vi "multitest.vi"   [LabVIEW 2015, in "SystemLink File Module tests.lvlib"]
uses:
  SystemLink File Module tests.lvlib
  module/configuration/SystemLink File configuration.lvclass
  <vilib>/Skyline/Tag/Wrapper/Wrapper_class/NI Skyline Tag.lvclass
  <vilib>/Skyline/Tag/Wrapper/Wrapper_class/Generate Tag Cluster (DBL).vi
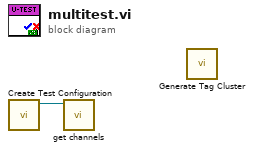
[diagram p0: block diagram]
diagram:
  n1 = call "Create Test Configuration.vi"() -> ("Module Configuration"=w1:refnum<class "SystemLink File configuration.lvclass">)  [unwired: 6 in, 5 out]
  n2 = call-dynamic "get channels.vi"("SystemLin Tag Module configuration in"=w1) -> ()  [unwired: 9 in, 2 out]
  n3 = call-poly <vilib>:"Generate Tag Cluster.vi"() -> ()  [unwired: 9 in, 3 out]
